vi "svl_Low Pass [Order 2] No State.vi"(6 "state info in":T1 {"y(n-2) state" format="%.2f"; "x(n-2) state" format="%.2f"; "y(n-1) state" format="%.2f"; "x(n-1) state" format="%.2f"}, 9 "reset":bool=TRUE, 10 "filter coefficients":cluster{"beta":dbl, "gamma":dbl, "alpha":dbl} {"alpha" format="%.2f"; "gamma" format="%.2f"; "beta" format="%.2f"}, 11 "Input stream":dbl[](array[numeric])) -> (3 "filtered signal":dbl[](array[numeric]), 4 "state info out":T1 {"y(n-2) state" format="%.2f"; "x(n-2) state" format="%.2f"; "y(n-1) state" format="%.2f"; "x(n-1) state" format="%.2f"})   [LabVIEW 2017, in "SoundVib_Integration.lvlib"]
uses:
  <vilib>/addons/Sound and Vibration/svt_Integration/SoundVib_Integration.lvlib
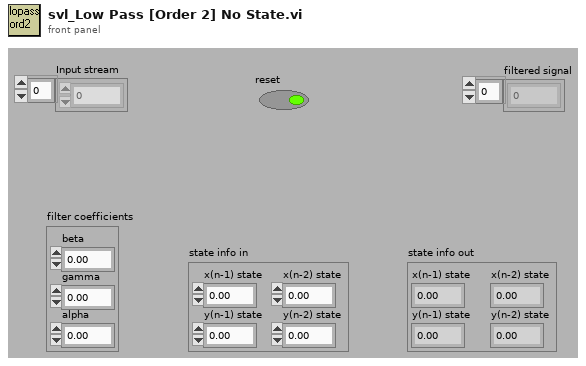
[diagram p1: front panel]
types:
  T1 = cluster{"x(n-1) state":dbl, "y(n-1) state":dbl, "x(n-2) state":dbl, "y(n-2) state":dbl}
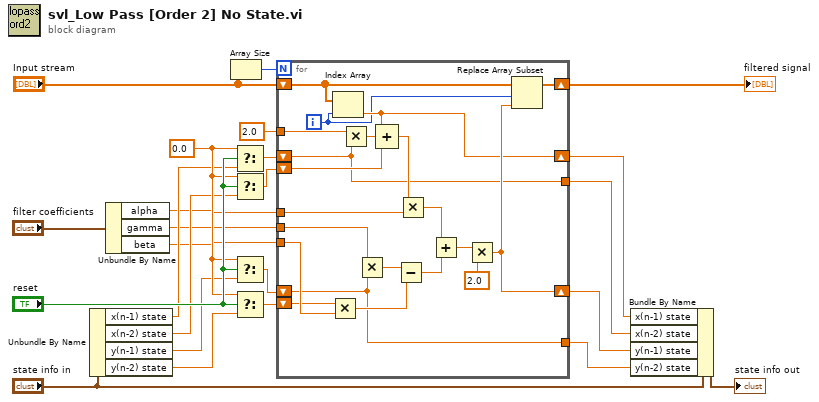
[diagram p0: block diagram]
diagram:
  w22 = 0.0 ("x")
  n1 = Unbundle By Name("state info in") -> ("x(n-1) state"=w11:dbl, "x(n-2) state"=w10:dbl, "y(n-1) state"=w20:dbl, "y(n-2) state"=w9:dbl)
  n2 = Unbundle By Name("filter coefficients") -> ("alpha"=w3:dbl, "gamma"=w4:dbl, "beta"=w5:dbl)
  n3 = Array Size(array="Input stream") -> (size(s)=w2:i32)
  n4 = Select(t=w22, s="reset", f=w11) -> (s? t:f=w14:dbl)
  n5 = Select(t=w22, s="reset", f=w10) -> (s? t:f=w13:dbl)
  n6 = Select(t=w22, s="reset", f=w20) -> (s? t:f=w15:dbl)
  n7 = Select(t=w22, s="reset", f=w9) -> (s? t:f=w12:dbl)
  n8 = for {
    N: w2 -> [_]
    shift-right: [w28] -> w19
    shift-left: w14 -> [w29]
    shift-left: w13 -> [w33]
    tunnel: 2.0 ("x") -> [w45]
    tunnel: w3 -> [w42]
    shift-right: [w34] -> w8
    shift-left: w15 -> [w32]
    shift-left: w12 -> [w31]
    tunnel: w4 -> [w30]
    tunnel: w5 -> [w38]
    tunnel: [w29] -> w18
    tunnel: [w32] -> w17
    shift-right: [w27] -> w21
    shift-left: "Input stream" -> [w25]
    i -> [w26]
    n9 = Multiply(x=w31, y=w38) -> (x*y=w37:dbl)
    n10 = Index Array(array=w25, index=w26) -> (element=w28:dbl)
    n11 = Multiply(x=w45, y=w29) -> (x*y=w44:dbl)
    n12 = Multiply(x=w30, y=w32) -> (x*y=w40:dbl)
    n13 = Compound Arithmetic op=ADD(w28, w44, w33) -> (w43:dbl)
    n14 = Subtract(x=w40, y=w37) -> (x-y=w39:dbl)
    n15 = Multiply(x=w43, y=w42) -> (x*y=w41:dbl)
    n16 = Add(x=w41, y=w39) -> (x+y=w36:dbl)
    n17 = Multiply(x=w36, y=2.0) -> (x*y=w34:dbl)
    n18 = Replace Array Subset(array=w25, new element=w34, index=w26) -> (w27:dbl[])
  }
  "filtered signal" <- w21
  n19 = Bundle By Name(cluster="state info in", "x(n-1) state"=w19, "x(n-2) state"=w18, "y(n-1) state"=w8, "y(n-2) state"=w17) -> (→"state info out":T1)
